vi "e.gate Example - HighSpeedPort Read Diagnostics.vi"() -> ()   [LabVIEW 2016]
uses:
  e.gate Diagnostic Interface Data.ctl
  e.gate Diagnostic Transport Data.ctl
  e.gate Diagnostic Variable Data.ctl
  e.gate Protocol Type.ctl
  e.gate HighSpeedPort Diagnostics Full.vi
panel:
  out "e.gate Variable Diagnostic Data":T1
  out "e.gate Transport Diagnostic Data":T2
  out "e.gate Interface Diagnostic Data":T3={"Interface Kind"=["Fieldbus", "Internal System", "Internal System", "ExternalUART", "ExternalUART", "ExternalUART"], "Interface Index"=[0, 0, 0, 0, 1, 2], "Cycles Count"=[280401, 280401, 280401, 280401, 14024, 280401], "Error Count"=[0, 0, 0, 0, 0, 0], "DeltaTimeS"=[1402.004973, 1402.004982, 1402.004982, 1402.004982, 1402.004983, 1402.004983]}
  out "error out":errorcluster
  in  "IP Address":string
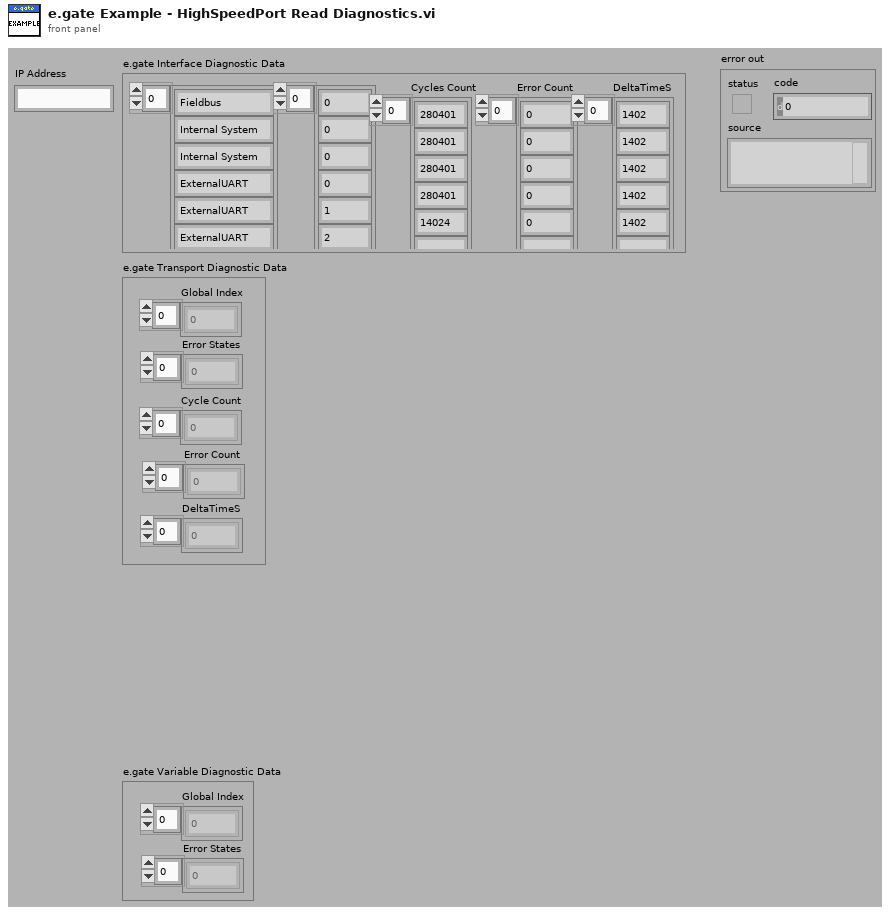
[diagram p1: front panel]
types:
  T1 = typedef "e.gate Diagnostic Variable Data.ctl" = cluster{"Global Index":i16[], "Error States":i16[]}
  T2 = typedef "e.gate Diagnostic Transport Data.ctl" = cluster{"Global Index":i16[], "Error States":i16[], "Cycle Count":i32[], "Error Count":i32[], "DeltaTimeS":dbl[]}
  T3 = typedef "e.gate Diagnostic Interface Data.ctl" = cluster{"Interface Kind":string[], "Interface Index":i16[], "Cycles Count":i32[], "Error Count":i32[], "DeltaTimeS":dbl[]}
  T4 = typedef "e.gate Protocol Type.ctl" = enum16{"ASCII", "HighspeedPort Online", "HighspeedPort Buffer", "eGateHighspeedPortDLL "}
  T5 = typedef "e.gate Configuration.ctl" = cluster{"connection ID":refnum<k5>, "IPAddress":string, "BufferIndex":i32, "StateMessage":string, "StateCode":i8, "HeaderSize":i32, "BufferSize":i32, "IsBigEndian":i32, "Version":i32, "ChannelCount":i32, "FrameLength":i32, "StartTime":dbl, "dActTimeToSecondFactor":dbl, "StartTimeToDayFactor":dbl, "BufferFillRate":dbl, "SampleRate":dbl, "ChannelData":T6[], "DecodeTimeFormat":string, "SummaryPath":string, "WithCheckSum":i32, "dActTimeDataType":T7, "MaxWriteCount":i32, "MaxReadCount":i32, "TempOffsetRead":i32, "TempLengthRead":i32, "Protocol":T4, "IsSupported":i32, "InputAccessList":i32[], "OutputAccessList":i32[], "DataSource":enum16{"CircleBuffer", "test.con Logger", "test.con Archive"}, "Modules":T8[], "DLL-Handle":T9}
  T6 = typedef "e.gate Channel Data.ctl" = cluster{"VariableName":string, "DataDirection":string, "DataType":string, "DataTypeIndex":T7, "Precision":i16, "FieldLengtht":i16, "ByteCount":i32, "Format":string, "Unit":string, "InputAccessOffset":i32, "OutputAccessOffset":i16, "InputAccessIndex":i16, "OutputAccessIndex":i16, "VarType":string}
  T7 = typedef "e.gate Data Type.ctl" = enum16{"NO", "BOOL", "SINT8", "USINT8", "SINT16", "USINT16", "SINT32", "USINT32", "FLOAT", "SET8", "SET16", "SET32", "DOUBLE", "SINT64", "USINT64", "SET64"}
  T8 = typedef "e.gate Module  Data.ctl" = cluster{"Type":string, "Location":string, "VariablesCount":i16, "UartIndex":i16, "Address":i16, "SystemOffset":i16}
  T9 = typedef "e.gateHSP_DLLhandle.ctl" = cluster{"clientInstance":i32, "connectionInstance":i32}
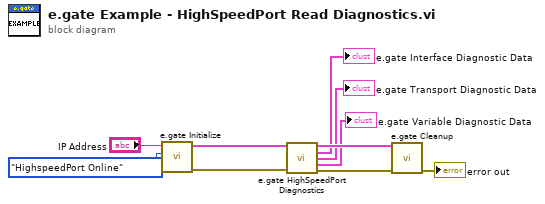
[diagram p0: block diagram]
diagram:
  n1 = call "e.gate Initialize.vi"("Protocol"=e.gate_Protocol_Type."HighspeedPort Online", "IP Address"="IP Address") -> ("error out"=w9:errorcluster, "e.gate Configuration"=w10:T5)  [unwired: 8 in]
  n2 = call-poly "e.gate HighSpeedPort Diagnostics.vi"("e.gate Configuration"=w10, "error in (no error)"=w9) -> ("e.gate Configuration out"=w8:T5, "e.gate Interface Diagnostic Data"=→"e.gate Interface Diagnostic Data":T3, "e.gate Transport Diagnostic Data"=→"e.gate Transport Diagnostic Data":T2, "e.gate Variable Diagnostic Data"=→"e.gate Variable Diagnostic Data":T1, "error out"=w7:errorcluster)  [unwired: 9 in]
  n3 = call "e.gate Cleanup.vi"("error in (no error)"=w7, "e.gate Configuration"=w8) -> ("error out"=→"error out":errorcluster)  [unwired: 9 in]
